vi "Open TCP Connection.vi"(8 "error in (no error)":errorcluster, 11 "Domino Laser module Class in":refnum<class "Domino Laser module Class.lvclass">) -> (0 "error out":errorcluster, 3 "Domino Laser module Class out":refnum<class "Domino Laser module Class.lvclass">)   [LabVIEW 2024, in "Domino LM.lvlib" / "Domino Laser module Class.lvclass"]
uses:
  CTRLS/Domino Laser module Class.lvclass
  CTRLS/Domino Laser module Class.lvclass/Domino Laser module Class.ctl
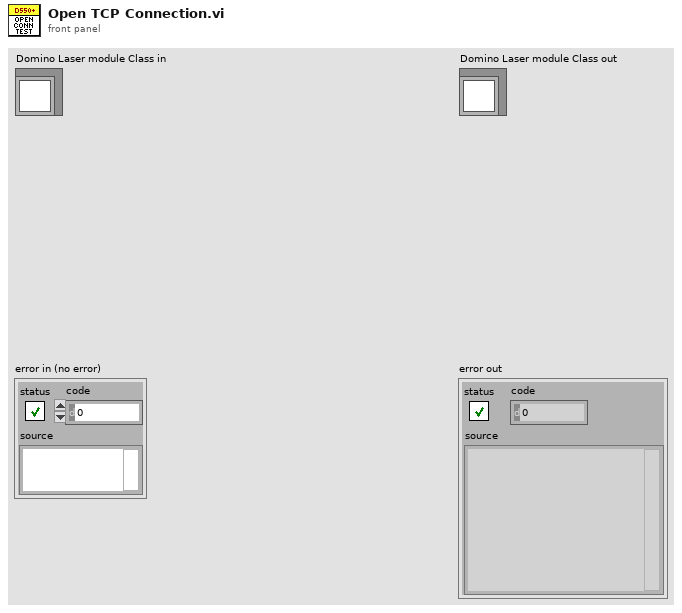
[diagram p1: front panel]
types:
  T1 = enum16{"Standard", "Buffered", "CRLF", "Immediate"}
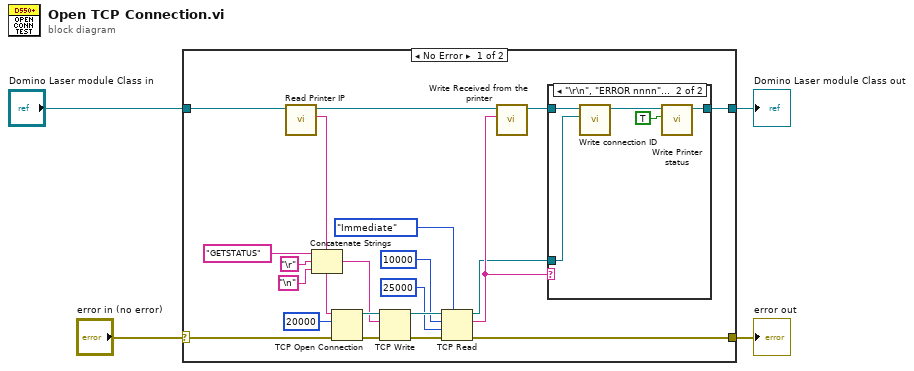
[diagram p0: block diagram]
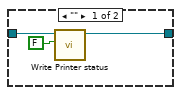
[diagram p2: hidden frame]
diagram:
  n1 = case shown="No Error" "error in (no error)" {
    selector: "error in (no error)" -> [w13 w35]
    tunnel: [w12 w35] -> w3
    tunnel: [w19 w34] -> w1
    tunnel: "Domino Laser module Class in" -> [w15 w34]
    frame No Error {
      n2 = call "Read Printer IP.vi"("Domino Laser module Class in"=w15) -> ("Printer IP"=w5:string, "Domino Laser module Class out"=w14:refnum<class "Domino Laser module Class.lvclass">)  [unwired: 8 in, 1 out]
      n3 = Concatenate Strings("GETSTATUS" ("data in"), "\r", "\n") -> (w8:string)
      n4 = TCP Open Connection(address=w5, remote port or service name=u16 20000, error in (no error)=w13) -> (connection ID=w22:refnum<k5>, error out=w23:errorcluster)  [unwired: 2 in]
      n5 = TCP Write(connection ID=w22, data in=w8, error in (no error)=w23) -> (connection ID out=w21:refnum<k5>, error out=w20:errorcluster)  [unwired: 1 in, 1 out]
      n6 = TCP Read(connection ID=w21, bytes to read=10000, error in (no error)=w20, 7:T1."Immediate" ("mode (standard)"), 9:25000 ("timeout ms (25000)")) -> (connection ID out=w16:refnum<k5>, data out=w18:string, error out=w12:errorcluster)
      n7 = call "Write Received from the printer.vi"("Received from the printer"=w18, "Domino Laser module Class in"=w14) -> ("Domino Laser module Class out"=w17:refnum<class "Domino Laser module Class.lvclass">)  [unwired: 8 in, 1 out]
      n8 = case shown="\"\\r\\n\", \"ERROR nnnn\", Default" w18 {
        tunnel: w17 -> [w26 w31]
        tunnel: [w28 w33] -> w19
        tunnel: w16 -> [_ w29]
        frame "" {
          n9 = call "Write Printer status.vi"("Printer status"=FALSE, "Domino Laser module Class in"=w26) -> ("Domino Laser module Class out"=w28:refnum<class "Domino Laser module Class.lvclass">)  [unwired: 8 in, 1 out]
        }
        frame "\r\n", "ERROR nnnn", Default {
          n10 = call "Write connection ID.vi"("connection ID"=w29, "Domino Laser module Class in"=w31) -> ("Domino Laser module Class out"=w30:refnum<class "Domino Laser module Class.lvclass">)  [unwired: 8 in, 1 out]
          n11 = call "Write Printer status.vi"("Printer status"=TRUE, "Domino Laser module Class in"=w30) -> ("Domino Laser module Class out"=w33:refnum<class "Domino Laser module Class.lvclass">)  [unwired: 8 in, 1 out]
        }
      }
    }
    frame Error {
    }
  }
  "error out" <- w3
  "Domino Laser module Class out" <- w1
